vi "Update.vi"(8 "error in (no error)":errorcluster, 10 "Message in":refnum<class "UpdateMessage.lvclass">, 11 "StageSPIM in":refnum<class "StageSPIM.lvclass">) -> (0 "error out":errorcluster, 3 "StageSPIM out":refnum<class "StageSPIM.lvclass">)   [LabVIEW 2012, in "StageSPIM.lvclass"]
doc: "The update method processes the command 'update'. \n\nThe command 'update' is used for receiving new values to be set to the private data of the class. This could be seen as a public set method for setting new parameters to the private class data."
uses:
  StageSPIM.lvclass
  <vilib>/Distrio/Murmex/UpdateMessage/UpdateMessage.lvclass
  StageSPIM.lvclass/StageSPIM.ctl
  <vilib>/Distrio/Murmex/Murmex/Murmex.lvclass
panel:
  # "This method is called when the UPDATE\ntrigger is sent. \n\nOverride this method when your component needs to\nrespond to this trigger. \n\nCall parent for proper implementation"
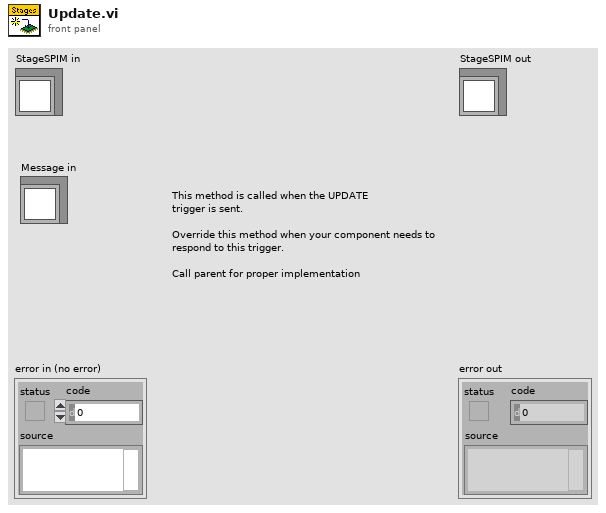
[diagram p1: front panel]
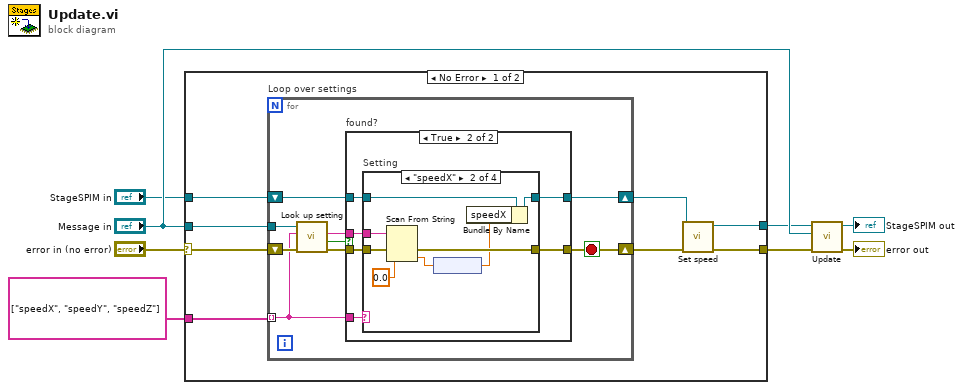
[diagram p0: block diagram]
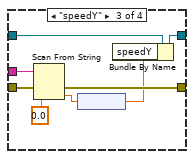
[diagram p4: hidden frame]
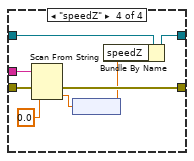
[diagram p5: hidden frame]
diagram:
  n1 = case shown="No Error" "error in (no error)" {
    selector: "error in (no error)" -> [w16 w60]
    tunnel: [w11 w60] -> w5
    tunnel: string[] ["speedX", "speedY", "speedZ"] ("key chains") -> [w15 _]
    tunnel: "Message in" -> [w14 _]
    tunnel: "StageSPIM in" -> [w13 w61]
    tunnel: [w9 w61] -> w1
    frame No Error {
      n2 = for "Loop over settings" {
        shift-right: [w17] -> w12
        shift-left: w16 -> [w25]
        tunnel: w15 -> [w19] mode=indexing
        tunnel: w14 -> [w24]
        shift-right: [w18] -> w10
        shift-left: w13 -> [w22]
        stop <- w17 stop-if-true
        n3 = call <vilib>:"Look up setting.vi"("error in (no error)"=w25, "tag name"=w19, "UpdateMessage in"=w24) -> ("error out"=w20:errorcluster, "found?"=w23:bool, "value"=w21:string)  [unwired: 5 in, 1 out]
        n4 = case "found?" shown="True" w23 {
          tunnel: w22 -> [w27 w31]
          tunnel: w21 -> [_ w32]
          tunnel: w20 -> [w26 w30]
          tunnel: w19 -> [_ w33]
          tunnel: [w27 w29] -> w18
          tunnel: [w26 w28] -> w17
          frame False {
          }
          frame True {
            n5 = case "Setting" shown="\"speedX\"" w33 {
              tunnel: w32 -> [_ w42 w46 w55]
              tunnel: w31 -> [w35 w41 w50 w58]
              tunnel: w30 -> [w34 w43 w51 w59]
              tunnel: [w35 w40 w49 w57] -> w29
              tunnel: [w34 w39 w47 w56] -> w28
              frame Default {
              }
              frame "speedX" {
                n6 = Scan From String(input string=w42, error in=w43, default 1=0.0 ("Settings_cluster.Power")) -> (error out=w39:errorcluster, output 1=w38:dbl)  [unwired: 2 in, 2 out]
                n7 = node(w38) -> (w37:dbl[unit])
                n8 = Bundle By Name(cluster=w41, "speedX"=w37) -> (w40:refnum<class "StageSPIM.lvclass">)
              }
              frame "speedY" {
                n9 = Scan From String(input string=w46, error in=w51, default 1=0.0 ("Settings_cluster.Power")) -> (error out=w47:errorcluster, output 1=w45:dbl)  [unwired: 2 in, 2 out]
                n10 = node(w45) -> (w44:dbl[unit])
                n11 = Bundle By Name(cluster=w50, "speedY"=w44) -> (w49:refnum<class "StageSPIM.lvclass">)
              }
              frame "speedZ" {
                n12 = Scan From String(input string=w55, error in=w59, default 1=0.0 ("Settings_cluster.Power")) -> (error out=w56:errorcluster, output 1=w54:dbl)  [unwired: 2 in, 2 out]
                n13 = node(w54) -> (w53:dbl[unit])
                n14 = Bundle By Name(cluster=w58, "speedZ"=w53) -> (w57:refnum<class "StageSPIM.lvclass">)
              }
            }
          }
        }
      }
      n15 = call-dynamic "Set speed.vi"("error in (no error)"=w12, "StageSPIM in"=w10) -> ("error out"=w11:errorcluster, "StageSPIM out"=w9:refnum<class "StageSPIM.lvclass">)  [unwired: 8 in]
    }
    frame Error {
    }
  }
  n16 = call-parent "Update.vi"("error in (no error)"=w5, "Message in"="Message in", "Murmex in"=w1) -> ("error out"=→"error out":errorcluster, "Murmex out"=→"StageSPIM out":refnum<class "StageSPIM.lvclass">)  [unwired: 7 in]
